vi "hmp4000 Open.vi"(8 "error in (no error)":errorcluster) -> (0 "error out":errorcluster)   [LabVIEW 2022 SP3]
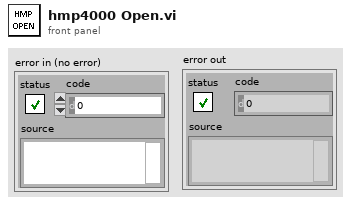
[diagram p1: front panel]
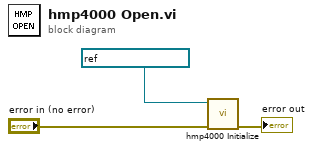
[diagram p0: block diagram]
diagram:
  n1 = call <instrlib>:"hmp4000 Initialize.vi"("error in (no error)"="error in (no error)", "VISA resource name"=refnum<visa-resource-name> "HMP4040_FTS2") -> ("error out"=→"error out":errorcluster)  [unwired: 8 in, 1 out]
